vi "Helper SubVI - Model Histogram.vi"(8 "error in (no error)":errorcluster, 9 "step size (Hz)":dbl=1.0, 10 "range (Hz)":dbl=1.0, 11 "freq (Hz)":dbl[][](array[numeric])) -> (0 "error out":errorcluster, 3 "Mode Histogram":cluster{cluster{dbl, dbl}[]}[](array[cluster]))   [LabVIEW 2023]
doc: "Forms a mode histrogram from the frequency array."
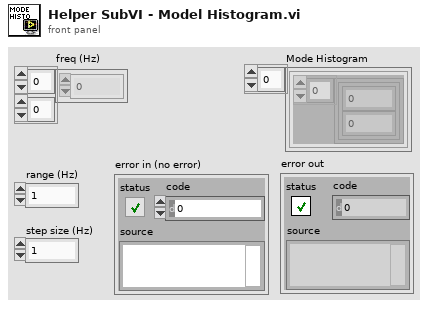
[diagram p1: front panel]
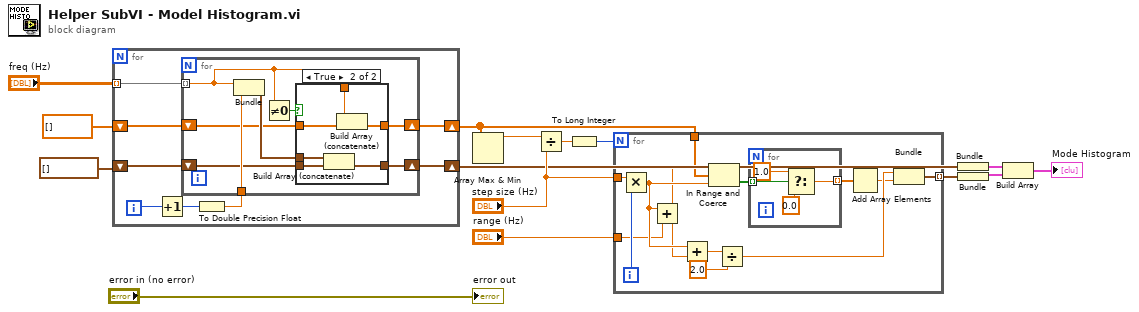
[diagram p0: block diagram]
diagram:
  n1 = for {
    tunnel: "freq (Hz)" -> [w23] mode=indexing
    shift-right: [w20] -> w8
    shift-left: cluster{dbl, dbl}[] [] -> [w21]
    shift-right: [w18] -> w3
    shift-left: dbl[] [] -> [w17]
    i -> [w22]
    n2 = Increment(x=w22) -> (x+1=w19:i32)
    n3 = To Double Precision Float(number=w19) -> (double precision float=w16:dbl)
    n4 = for {
      tunnel: w23 -> [w24] mode=indexing
      tunnel: w16 -> [w31]
      shift-right: [w26] -> w20
      shift-left: w21 -> [w29]
      shift-right: [w27] -> w18
      shift-left: w17 -> [w28]
      n5 = Bundle(w24, w31) -> (w30:cluster{dbl, dbl})  [unwired: 1 out]
      n6 = Not Equal To 0?(x=w24) -> (x != 0?=w25:bool)
      n7 = case shown="True" w25 {
        tunnel: w30 -> [_ w39]
        tunnel: w29 -> [w32 w38]
        tunnel: w24 -> [_ w37]
        tunnel: w28 -> [w33 w36]
        tunnel: [w33 w35] -> w27
        tunnel: [w32 w34] -> w26
        frame False {
        }
        frame True {
          n8 = Build Array (concatenate)(w39, w38) -> (w34:cluster{dbl, dbl}[])
          n9 = Build Array (concatenate)(w37, w36) -> (w35:dbl[])
        }
      }
    }
  }
  n10 = Array Max & Min(array=w3) -> (max value=w12:dbl)  [unwired: 3 out]
  n11 = Divide(x=w12, y="step size (Hz)") -> (x/y=w11:dbl)
  n12 = To Long Integer(number=w11) -> (32bit integer=w10:i32)
  n13 = for {
    N: w10 -> [_]
    tunnel: "step size (Hz)" -> [w52]
    tunnel: w3 -> [w50]
    tunnel: [w43] -> w7 mode=indexing
    tunnel: "range (Hz)" -> [w40]
    i -> [w51]
    n14 = Multiply(x=w52, y=w51) -> (x*y=w42:dbl)
    n15 = Add(x=w42, y=w40) -> (x+y=w41:dbl)
    n16 = Add(x=w42, y=w41) -> (x+y=w47:dbl)
    n17 = In Range and Coerce(upper limit=w41, x=w50, lower limit=w42) -> (In Range?=w49:bool[])  [unwired: 1 out]
    n18 = Divide(x=w47, y=2.0) -> (x/y=w45:dbl)
    n19 = for {
      tunnel: w49 -> [w56] mode=indexing
      tunnel: [w53] -> w48 mode=indexing
      n20 = Select(t=1.0, s=w56, f=0.0) -> (s? t:f=w53:dbl)
    }
    n21 = Add Array Elements(numeric array=w48) -> (sum=w44:dbl)
    n22 = Bundle(w45, "f"=w44) -> (w43:cluster{dbl, "f":dbl})  [unwired: 1 out]
  }
  n23 = Bundle(w8) -> (w6:cluster{cluster{dbl, dbl}[]})  [unwired: 1 in]
  n24 = Bundle(w7) -> (w5:cluster{cluster{dbl, "f":dbl}[]})  [unwired: 1 in]
  n25 = Build Array(w6, w5) -> (→"Mode Histogram":cluster{cluster{dbl, "f":dbl}[]}[])
  "error out" <- "error in (no error)"
